vi "Write Transfer Buffer.vi"(8 "error in (no error)":errorcluster, 9 "data":string, 10 "Transfer":refnum<class "Transfer.lvclass">, 11 "UDP Transceiver in":refnum<class "UDP Transceiver.lvclass">) -> (0 "error out":errorcluster, 3 "UDP Transceiver out":refnum<class "UDP Transceiver.lvclass">)   [LabVIEW 2017, in "UDP Transceiver.lvclass"]
uses:
  UDP Transceiver.lvclass
  Classes/Transfer/Transfer.lvclass
  Classes/Buffer/Write Buffer 1D U8.vi
  Throw Size Mismatch Error.vi
  Classes/Buffer/Buffer.lvclass
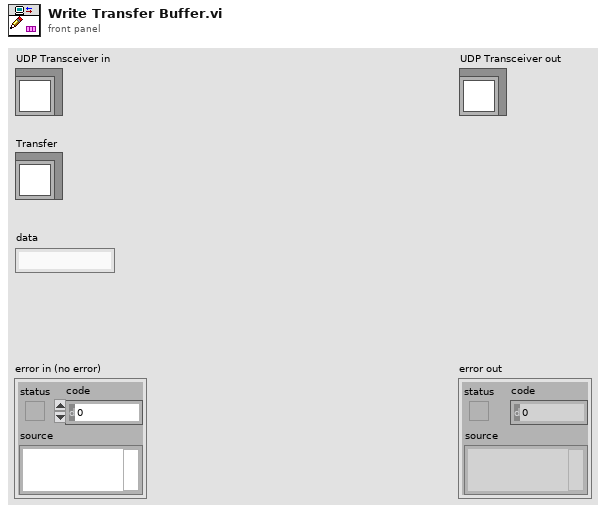
[diagram p1: front panel]
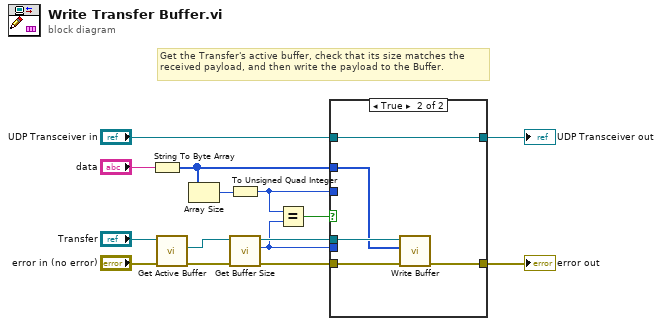
[diagram p0: block diagram]
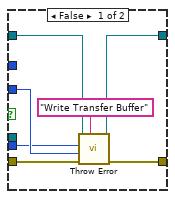
[diagram p2: hidden frame]
diagram:
  # "Get the Transfer's active buffer, check that its size matches the received payload, and then write the payload to the Buffer."
  n1 = String To Byte Array(string="data") -> (unsigned byte array=w12:u8[])
  n2 = call "Get Active Buffer.vi"("error in (no error)"="error in (no error)", "Transfer in"="Transfer") -> ("error out"=w2:errorcluster, "Buffer"=w1:refnum<class "Buffer.lvclass">)  [unwired: 7 in, 1 out]
  n3 = Array Size(array=w12) -> (size(s)=w14:i32)
  n4 = To Unsigned Quad Integer(1:w14) -> (0:w9:u64)
  n5 = call "Get Buffer Size.vi"("Buffer in"=w1) -> ("buffer size"=w10:u64, "Buffer out"=w13:refnum<class "Buffer.lvclass">)  [unwired: 9 in]
  n6 = Equal?(x=w9, y=w10) -> (x = y?=w11:bool)
  n7 = case shown="True" w11 {
    tunnel: w13 -> [_ w26]
    tunnel: w2 -> [w21 w25]
    tunnel: [w20 w24] -> w8
    tunnel: w12 -> [_ w22]
    tunnel: "UDP Transceiver in" -> [w19 w23]
    tunnel: [w18 w23] -> w7
    tunnel: w10 -> [w16 _]
    tunnel: w9 -> [w17 _]
    frame False {
      n8 = call-poly "Throw Error.vi"("source vi name"="Write Transfer Buffer", "error in (no error)"=w21, "actual size"=w17, "expected size"=w16, "UDP in"=w19) -> ("error out"=w20:errorcluster, "UDP out"=w18:refnum<class "UDP Transceiver.lvclass">)  [unwired: 5 in]
    }
    frame True {
      n9 = call-poly "Write Buffer.vi"("error in (no error)"=w25, "src array in"=w22, "Buffer in"=w26) -> ("error out"=w24:errorcluster)  [unwired: 5 in, 3 out]
    }
  }
  "error out" <- w8
  "UDP Transceiver out" <- w7
